vi "Execute State.vi"(8 "error in (no error)":errorcluster, 9 "Data":variant, 10 "State":string, 11 "ExampleSimpleRootModel in":refnum<class "SimpleRootModel.lvclass">) -> (0 "error out":errorcluster, 3 "ExampleSimpleRootModel out":refnum<class "SimpleRootModel.lvclass">)   [LabVIEW 2020, in "MVAExamples.lvlib" / "SimpleRootModel.lvclass"]
uses:
  SimpleRootModel.lvclass
  SimpleRootModel.lvclass/SimpleRootModel.ctl
  modules/mva-core/Source/IObserver/IObserver/IObserver.lvclass/IObserver.ctl
  modules/mva-core/Source/IModel/IModel/IModel.lvclass/IModel.ctl
  modules/mva-core/Source/IMediator/PublishRequest/PublishRequest.lvclass/PublishRequest.ctl
  modules/mva-core/Source/IMediator/IMediator Messages/Publish Msg/Publish Msg.lvclass/Publish Msg.ctl
  modules/composed-af-messages/Source/RoundTripMessage/RoundTripMessage.lvclass/RoundTripMessage.ctl
  <vilib>/ActorFramework/Message Enqueuer/Message Enqueuer.lvclass/Message Enqueuer.ctl
  modules/mva-core/Source/IMediator/IMediator Messages/Publish Msg/Send Pre-Addressed Publish.vi
  modules/mva-core/Source/IObserver/IObserver/Read Unique ID.vi
  modules/mva-core/Source/IMediator/PublishRequest/Pack Publish Request.vi
  modules/composed-af-messages/Source/RoundTripMessage/Return Round-Trip Message.vi
  <vilib>/ActorFramework/Message Enqueuer/Enqueue.vi
  modules/mva-core/Source/IModel/IModel/IModel.lvclass
  modules/mva-core/Source/IMediator/IMediator Messages/Publish Msg/Publish Msg.lvclass
  modules/composed-af-messages/Source/RoundTripMessage/RoundTripMessage.lvclass
  C:/Program Files/National Instruments/LabVIEW 2020/vi.lib/ActorFramework/Message/Message.lvclass
  <vilib>/Utility/error.llb/Error Cluster From Error Code.vi
  <vilib>/ActorFramework/Message Priority Queue/Priority Enqueue.vi
  modules/mva-core/Source/IMediator/PublishRequest/PublishRequest.lvclass
  C:/Program Files/National Instruments/LabVIEW 2020/vi.lib/ActorFramework/Actor/Actor.lvclass
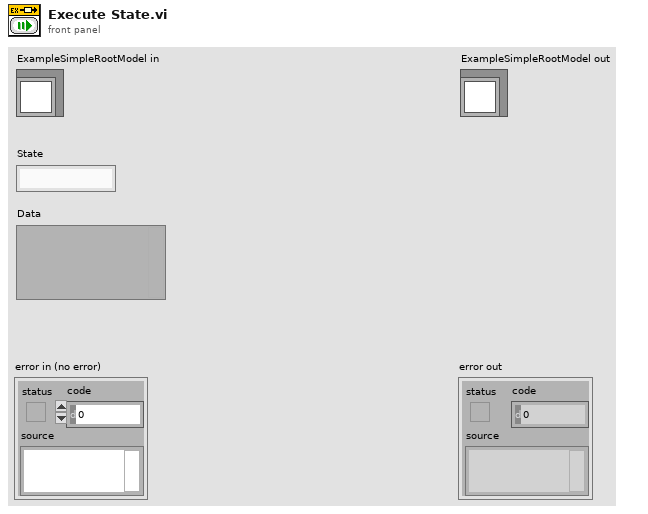
[diagram p1: front panel]
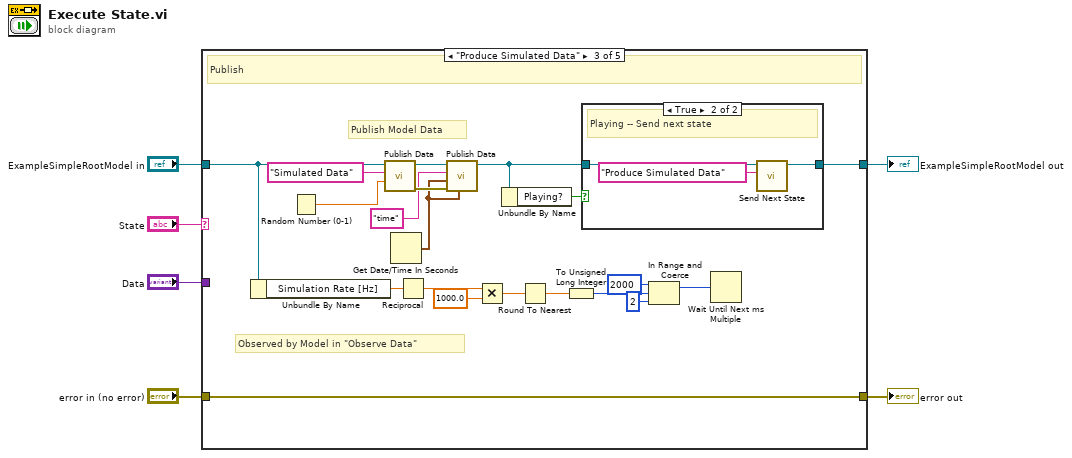
[diagram p0: block diagram]
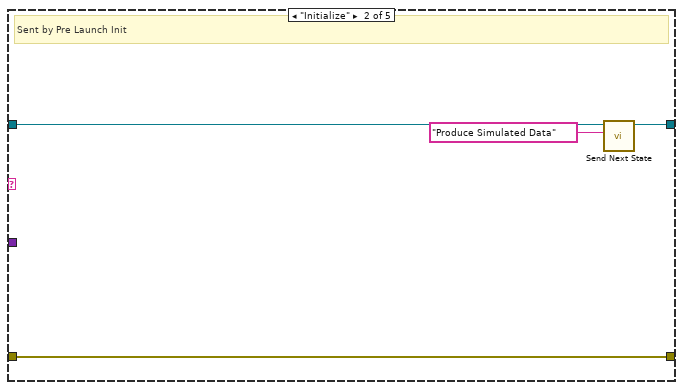
[diagram p3: hidden frame]
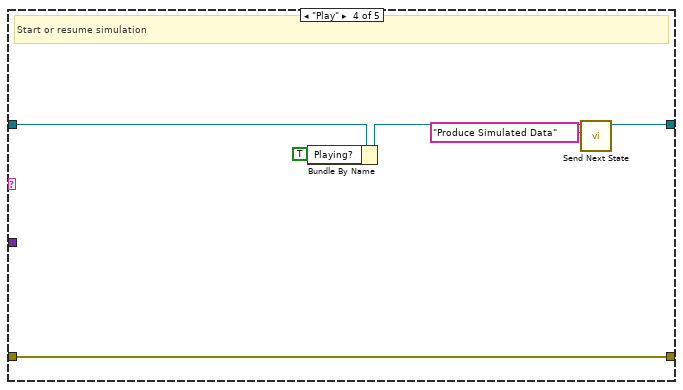
[diagram p5: hidden frame]
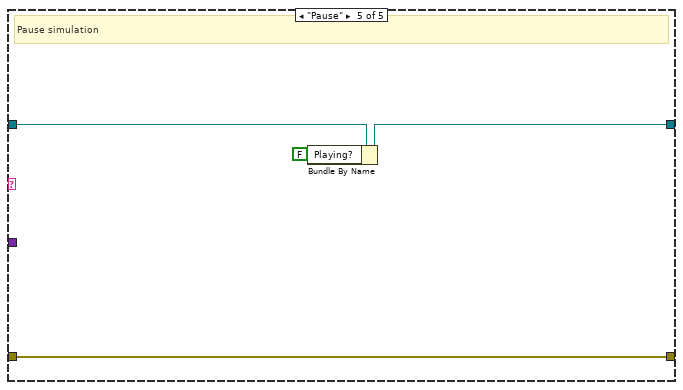
[diagram p6: hidden frame]
diagram:
  n1 = case shown="\"Produce Simulated Data\"" "State" {
    tunnel: [w7 w12 w32 w39 w43] -> w5
    tunnel: [w8 w10 w31 w38 w45] -> w3
    tunnel: "ExampleSimpleRootModel in" -> [w8 w11 w29 w42 w46]
    tunnel: "error in (no error)" -> [w7 w12 w32 w39 w43]
    tunnel: "Data" -> [_ _ _ _ _]
    frame Default {
      # "Unknown State Request"
    }
    frame "Initialize" {
      # "Sent by Pre Launch Init"
      n2 = call "Send Next State.vi"("State"="Produce Simulated Data", "ExampleSimpleRootModel in"=w11) -> ("ExampleSimpleRootModel out"=w10:refnum<class "SimpleRootModel.lvclass">)  [unwired: 8 in, 1 out]
    }
    frame "Produce Simulated Data" {
      # "Publish Model Data"
      # "Observed by Model in \"Observe Data\""
      # "Publish"
      n3 = Unbundle By Name(w29) -> ("Simulation Rate [Hz]"=w28:dbl)
      n4 = Random Number (0-1)() -> (number: 0 to 1=w18:dbl)
      n5 = call "Publish Data.vi"("Data to Publish"=w18, "Datum Name"="Simulated Data", "IModel in"=w29) -> ("error out"=w16:errorcluster, "IModel out"=w17:refnum<class "SimpleRootModel.lvclass">)  [unwired: 7 in]
      n6 = Get Date/Time In Seconds() -> (seconds since 1Jan1904=w13:timestamp)
      n7 = Reciprocal(x=w28) -> (1/x=w27:dbl)
      n8 = call "Publish Data.vi"("Publish Time (Use Current Time)"=w13, "error in (no error)"=w16, "Data to Publish"=w13, "Datum Name"="time", "IModel in"=w17) -> ("IModel out"=w15:refnum<class "SimpleRootModel.lvclass">)  [unwired: 5 in, 1 out]
      n9 = Multiply(x=w27, y=1000.0) -> (x*y=w25:dbl)
      n10 = Unbundle By Name(w15) -> ("Playing?"=w19:bool)
      n11 = Round To Nearest(number=w25) -> (nearest integer value=w23:dbl)
      n12 = To Unsigned Long Integer(number=w23) -> (unsigned 32bit integer=w24:u32)
      n13 = case shown="True" w19 {
        tunnel: [w33 w36] -> w31
        tunnel: w15 -> [w33 w34]
        frame False {
          # "Paused -- Stop sending message to self"
        }
        frame True {
          # "Playing -- Send next state"
          n14 = call "Send Next State.vi"("State"="Produce Simulated Data", "ExampleSimpleRootModel in"=w34) -> ("ExampleSimpleRootModel out"=w36:refnum<class "SimpleRootModel.lvclass">)  [unwired: 8 in, 1 out]
        }
      }
      n15 = In Range and Coerce(upper limit=u32 2000, x=w24, lower limit=u32 2) -> (coerced(x)=w22:u32)  [unwired: 1 out]
      n16 = Wait Until Next ms Multiple(millisecond multiple=w22) -> ()  [unwired: 1 out]
    }
    frame "Play" {
      # "Start or resume simulation"
      n17 = Bundle By Name(cluster=w42, "Playing?"=TRUE ("Play?")) -> (w41:refnum<class "SimpleRootModel.lvclass">)
      n18 = call "Send Next State.vi"("State"="Produce Simulated Data", "ExampleSimpleRootModel in"=w41) -> ("ExampleSimpleRootModel out"=w38:refnum<class "SimpleRootModel.lvclass">)  [unwired: 8 in, 1 out]
    }
    frame "Pause" {
      # "Pause simulation"
      n19 = Bundle By Name(cluster=w46, "Playing?"=FALSE ("Play?")) -> (w45:refnum<class "SimpleRootModel.lvclass">)
    }
  }
  "error out" <- w5
  "ExampleSimpleRootModel out" <- w3
